vi "FeedbackDecode_GenRandBlockIdxs2.vi"(0 "Mode":enum16{"Selected", "Block", "Random"}(ring), 1 "Reset":bool, 2 "NumTrials":dbl, 3 "NumIdxs":dbl, 4 "CurrIdx":dbl) -> (5 "RandIdx":dbl, 6 "Perc":dbl)   [LabVIEW 2020]
uses:
  <vilib>/imath/engines/lvmath2/RunTimeEngine/RangeToken/NIMS_Range.vi
  <instcachedir>/0/NIMS_Range_913EBD8295F041DB898D90A83F67761F.lvgen/NIMS_Range_913EBD8295F041DB898D90A83F67761F_000.vi
  <vilib>/imath/engines/lvmath2/RunTimeEngine/BuiltInFunctions/repeatmx/NIMS_repeatmx(GM, I32, I32).vi
  <instcachedir>/0/NIMS_repeatmx(GM, I32, I32)_32F7F84A1794440B83929A05B70BBBEE.lvgen/NIMS_repeatmx(GM, I32, I32)_32F7F84A1794440B83929A05B70BBBEE_000.vi
  <vilib>/imath/engines/lvmath2/RunTimeEngine/BuiltInFunctions/reshapemx/NIMS_[GV]_reshapemx.vi
  <instcachedir>/0/NIMS_[GV]_reshapemx_116A7F60707440F78CB0D64335A3F73C.lvgen/NIMS_[GV]_reshapemx_116A7F60707440F78CB0D64335A3F73C_000.vi
  <vilib>/imath/engines/lvmath2/RunTimeEngine/ErrorHandling/NIMS_Create Error From Enums.vi
  <vilib>/imath/engines/lvmath2/RunTimeEngine/BuiltInFunctions/length/NIMS_length(GV).vi
  <instcachedir>/0/NIMS_length(GV)_08A3D13377FD4E4B96F5795FBF3698FA.lvgen/NIMS_length(GV)_08A3D13377FD4E4B96F5795FBF3698FA_000.vi
  <vilib>/imath/engines/lvmath2/RunTimeEngine/BuiltInFunctions/randpermutation/NIMS_randpermutation.vi
  <vilib>/imath/engines/lvmath2/RunTimeEngine/IndexRead/NIMS V(V).vi
  <instcachedir>/0/NIMS V(V)_298D9CB7BFEB42B8BC8D9C3C28AE8C70.lvgen/NIMS V(V)_298D9CB7BFEB42B8BC8D9C3C28AE8C70_000.vi
  <vilib>/imathl/engines/lvmath/Functions/Error Handling/Create Error.vi
  <vilib>/imath/engines/lvmath2/RunTimeEngine/NodeEndStatement/NIMS_NodeEndStatement_Output.vi
  <instcachedir>/0/NIMS_NodeEndStatement_Output_53EC0D466D134D7ABD903AC30B43404B.lvgen/NIMS_NodeEndStatement_Output_53EC0D466D134D7ABD903AC30B43404B_005.vi
  <vilib>/imath/engines/lvmath2/RunTimeEngine/ErrorHandling/NIMS_Finalize Error.vi
panel:
  out "IdxArray":dbl[](array[numeric])
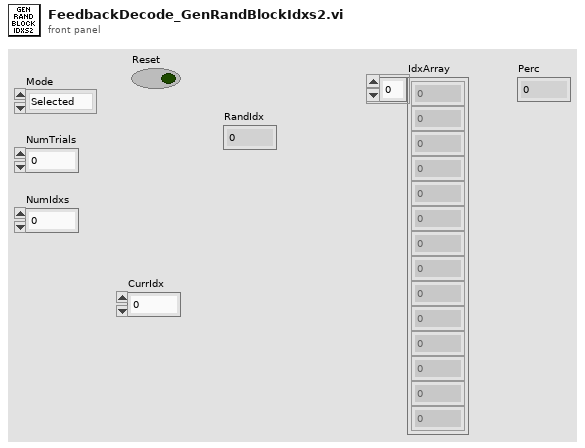
[diagram p1: front panel]
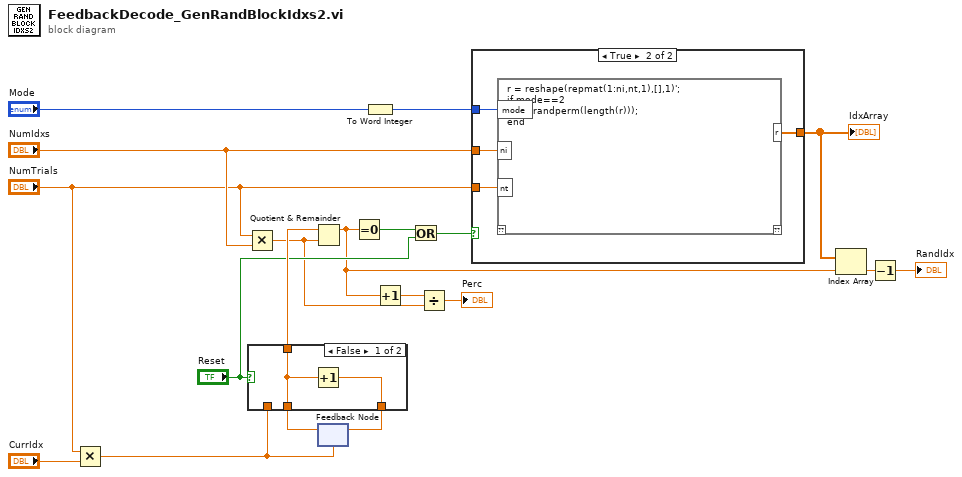
[diagram p0: block diagram]
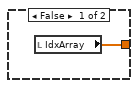
[diagram p3: hidden frame]
diagram:
  n1 = Multiply(x="NumTrials", y="CurrIdx") -> (x*y=w11:dbl)
  n2 = Multiply(x="NumTrials", y="NumIdxs") -> (x*y=w2:dbl)
  n3 = feedback #1(w11) -> (w16:dbl)
  n4 = case shown="False" "Reset" {
    tunnel: [w21 w22] -> w19
    tunnel: w16 -> [w20 _]
    tunnel: [w20 w22] -> w13
    tunnel: w11 -> [_ w22]
    frame False {
      n5 = Increment(x=w20) -> (x+1=w21:dbl)
    }
    frame True {
    }
  }
  n6 = Quotient & Remainder(x=w13, y=w2) -> (x-y*floor(x/y)=w4:dbl)  [unwired: 1 out]
  n7 = feedback-in #1(w19) -> ()
  n8 = Equal To 0?(x=w4) -> (x = 0?=w9:bool)
  n9 = To Word Integer(number="Mode") -> (16bit integer=w5:i16)
  n10 = Increment(x=w4) -> (x+1=w3:dbl)
  n11 = Or(x=w9, y="Reset") -> (x .or. y?=w7:bool)
  n12 = Divide(x=w3, y=w2) -> (x/y=→"Perc":dbl)
  n13 = case shown="True" w7 {
    tunnel: [w23 w27] -> w17
    tunnel: w5 -> [_ w26]
    tunnel: "NumIdxs" -> [_ w25]
    tunnel: "NumTrials" -> [_ w24]
    frame False {
      n14 = local read "IdxArray"() -> (w23:dbl[])
    }
    frame True {
      n15 = mathscript code="r = reshape(repmat(1:ni,nt,1),[],1)';\nif mode==2\nr = r(randperm(length(r)));\nend"("ni"=w25, "mode"=w26, "nt"=w24) -> ("r"=w27:dbl[])  [unwired: 1 in, 1 out]
    }
  }
  "IdxArray" <- w17
  n16 = Index Array(array=w17, index=w4) -> (element=w15:dbl)
  n17 = Decrement(x=w15) -> (x-1=→"RandIdx":dbl)
